vi "CreateTexture.vi"(4 "Pixel Format":T1=enum."SDL_PIXELFORMAT_RGBA8888", 6 "Texture Access":T2, 8 "No Error":errorcluster, 9 "h":i32, 10 "w":i32, 11 "Renderer [SDL_Renderer *]":T3 format="%.0x") -> (0 "error out":errorcluster, 3 "Texture [SDL_Texture *]":T4 format="%.0x")   [LabVIEW 2026, in "SDL3.lvlib" / "Render.lvlib"]
doc: "<B>Summary</B>\nCreate a texture for a rendering context.\n\n<B>Remarks</B>\nThe contents of a texture when first created are not defined."
uses:
  Render.lvlib
  TextureAccess-enum.ctl
  Pixels/PixelFormat--enum.ctl
  <vilib>/Utility/error.llb/Error Cluster From Error Code.vi
  Error/Error.lvlib
  Pixels/Pixels.lvlib
  Lib/SDL3.dll
  SDL_Renderer--pointer.ctl
  SDL_Texture--pointer.ctl
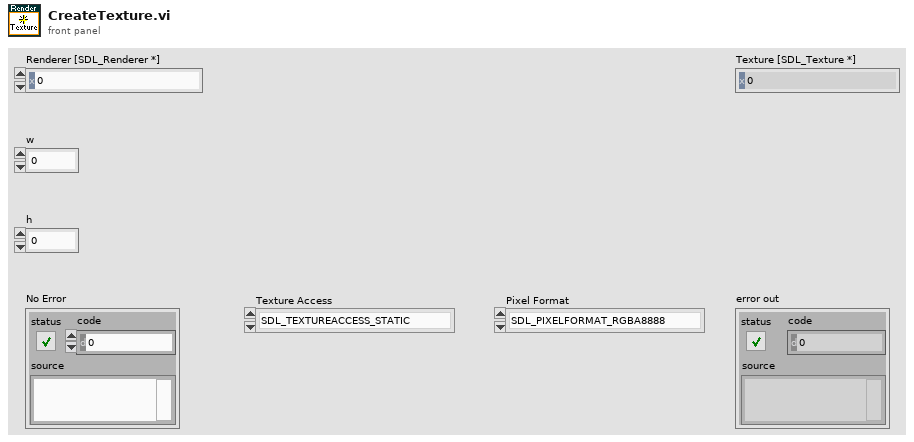
[diagram p1: front panel]
types:
  T1 = typedef "SDL3.lvlib/Pixels.lvlib/PixelFormat--enum.ctl" = enum32{"SDL_PIXELFORMAT_UNKNOWN", "SDL_PIXELFORMAT_INDEX1LSB", "SDL_PIXELFORMAT_INDEX1MSB", "SDL_PIXELFORMAT_INDEX2LSB", "SDL_PIXELFORMAT_INDEX2MSB", "SDL_PIXELFORMAT_INDEX4LSB", "SDL_PIXELFORMAT_INDEX4MSB", "SDL_PIXELFORMAT_INDEX8", "SDL_PIXELFORMAT_RGB332", "SDL_PIXELFORMAT_XRGB4444", "SDL_PIXELFORMAT_XBGR4444", "SDL_PIXELFORMAT_XRGB1555", "SDL_PIXELFORMAT_XBGR1555", "SDL_PIXELFORMAT_ARGB4444", "SDL_PIXELFORMAT_RGBA4444", "SDL_PIXELFORMAT_ABGR4444", "SDL_PIXELFORMAT_BGRA4444", "SDL_PIXELFORMAT_ARGB1555", "SDL_PIXELFORMAT_RGBA5551", "SDL_PIXELFORMAT_ABGR1555", "SDL_PIXELFORMAT_BGRA5551", "SDL_PIXELFORMAT_RGB565", "SDL_PIXELFORMAT_BGR565", "SDL_PIXELFORMAT_RGB24", "SDL_PIXELFORMAT_BGR24", "SDL_PIXELFORMAT_XRGB8888", "SDL_PIXELFORMAT_RGBX8888", "SDL_PIXELFORMAT_XBGR8888", "SDL_PIXELFORMAT_BGRX8888", "SDL_PIXELFORMAT_ARGB8888", "SDL_PIXELFORMAT_RGBA8888", "SDL_PIXELFORMAT_ABGR8888", "SDL_PIXELFORMAT_BGRA8888", "SDL_PIXELFORMAT_XRGB2101010", "SDL_PIXELFORMAT_XBGR2101010", "SDL_PIXELFORMAT_ARGB2101010", "SDL_PIXELFORMAT_ABGR2101010", "SDL_PIXELFORMAT_RGB48", "SDL_PIXELFORMAT_BGR48", "SDL_PIXELFORMAT_RGBA64", "SDL_PIXELFORMAT_ARGB64", "SDL_PIXELFORMAT_BGRA64", "SDL_PIXELFORMAT_ABGR64", "SDL_PIXELFORMAT_RGB48_FLOAT", "SDL_PIXELFORMAT_BGR48_FLOAT", "SDL_PIXELFORMAT_RGBA64_FLOAT", "SDL_PIXELFORMAT_ARGB64_FLOAT", "SDL_PIXELFORMAT_BGRA64_FLOAT", "SDL_PIXELFORMAT_ABGR64_FLOAT", "SDL_PIXELFORMAT_RGB96_FLOAT", "SDL_PIXELFORMAT_BGR96_FLOAT", "SDL_PIXELFORMAT_RGBA128_FLOAT", "SDL_PIXELFORMAT_ARGB128_FLOAT", "SDL_PIXELFORMAT_BGRA128_FLOAT", "SDL_PIXELFORMAT_ABGR128_FLOAT", "SDL_PIXELFORMAT_YV12", "SDL_PIXELFORMAT_IYUV", "SDL_PIXELFORMAT_YUY2", "SDL_PIXELFORMAT_UYVY", "SDL_PIXELFORMAT_YVYU", "SDL_PIXELFORMAT_NV12", "SDL_PIXELFORMAT_NV21", "SDL_PIXELFORMAT_P010", "SDL_PIXELFORMAT_EXTERNAL_OES"}
  T2 = typedef "SDL3.lvlib/Render.lvlib/TextureAccess-enum.ctl" = enum32{"SDL_TEXTUREACCESS_STATIC", "SDL_TEXTUREACCESS_STREAMING", "SDL_TEXTUREACCESS_TARGET"}
  T3 = typedef "SDL3.lvlib/Render.lvlib/SDL_Renderer--pointer.ctl" = i64
  T4 = typedef "SDL3.lvlib/Render.lvlib/SDL_Texture--pointer.ctl" = i64
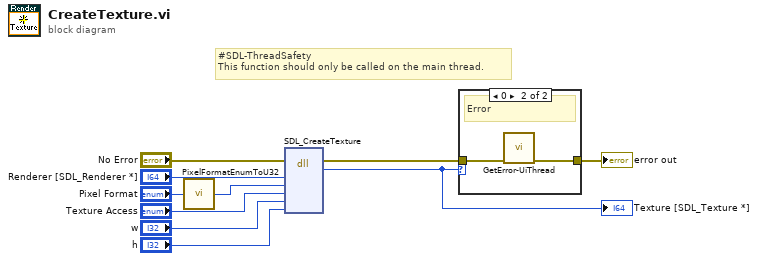
[diagram p0: block diagram]
diagram:
  # "#SDL-ThreadSafety\nThis function should only be called on the main thread."
  n1 = call "PixelFormatEnumToU32.vi"("PixelFormat--enum"="Pixel Format") -> ("PixelFormat"=w1:u32)
  n2 = dll-call lib="C:/Users/saukko/Dev/LV-SDL3/Sources/SDL3/Lib/SDL3.*" fn="SDL_CreateTexture"(error in="No Error", "renderer"="Renderer [SDL_Renderer *]", "pixel_format"=w1, "texture_access"="Texture Access", "w"="w", "h"="h") -> (error out=w2:errorcluster, "return type"=w6:i64)  [unwired: 7 in, 1 out]
  "Texture [SDL_Texture *]" <- w6
  n3 = case shown="0" w6 {
    tunnel: w2 -> [w11 w13]
    tunnel: [w11 w12] -> w9
    frame Default {
      # "Ok"
    }
    frame 0 {
      # "Error"
      n4 = call "GetError-UiThread.vi"("No Error"=w13) -> ("error out"=w12:errorcluster)  [unwired: 10 in]
    }
  }
  "error out" <- w9
